vi "GetPPLPath_VisionAnalysis.vi"(11 "FuncName":string) -> (2 "file or folder exists?":bool, 3 "appended path":path)   [LabVIEW 2015]
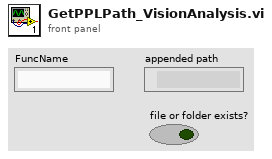
[diagram p1: front panel]
types:
  T1 = enum32{"invalid app kind", "Development System", "Run Time System", "Student Edition", "Embedded LabVIEW", "Evaluation", "Custom"}
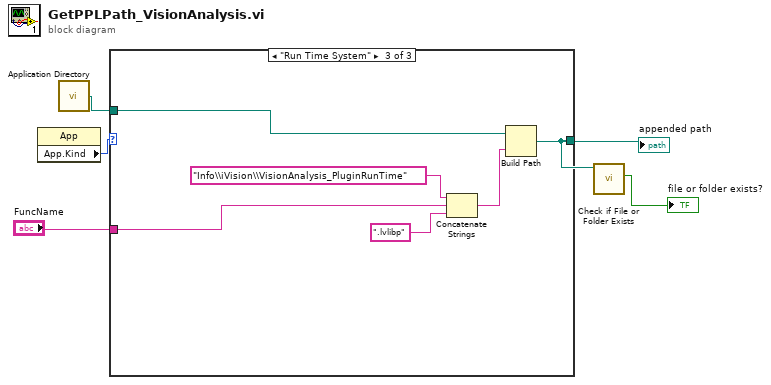
[diagram p0: block diagram]
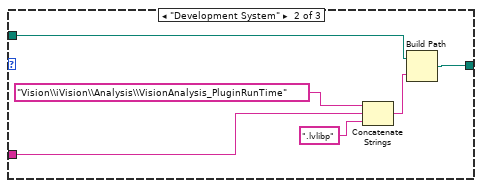
[diagram p3: hidden frame]
diagram:
  n1 = property class="App"() -> ("App.Kind"=w5:T1)  [unwired: 2 in, 2 out]
  n2 = call <vilib>:"Application Directory.vi"() -> ("Application Directory"=w4:path)
  n3 = case shown="\"Run Time System\"" w5 {
    tunnel: [_ w11 w17] -> w2
    tunnel: w4 -> [_ w7 w13]
    tunnel: "FuncName" -> [_ w10 w15]
    frame "invalid app kind", Default {
    }
    frame "Development System" {
      n4 = Concatenate Strings("Vision\\iVision\\Analysis\\VisionAnalysis_PluginRunTime" ("name or relative path"), w10, ".lvlibp") -> (w9:string)
      n5 = Build Path(base path=w7, name or relative path=w9) -> (appended path=w11:path)
    }
    frame "Run Time System" {
      n6 = Concatenate Strings("Info\\iVision\\VisionAnalysis_PluginRunTime" ("name or relative path"), w15, ".lvlibp") -> (w14:string)
      n7 = Build Path(base path=w13, name or relative path=w14) -> (appended path=w17:path)
    }
  }
  "appended path" <- w2
  n8 = call <vilib>:"Check if File or Folder Exists.vi"("path"=w2) -> ("file or folder exists?"=→"file or folder exists?":bool)  [unwired: 8 in, 2 out]
